vi "Credito Reset.vi"(8 "error in (no error)":errorcluster, 11 "USD Actor in":refnum<class "USD Actor.lvclass">) -> (0 "error out":errorcluster, 3 "USD Actor out":refnum<class "USD Actor.lvclass">)   [LabVIEW 2020, in "USD Actor.lvlib" / "USD Actor.lvclass"]
uses:
  USD Actor.lvclass
  USD Actor.lvclass/USD Actor.ctl
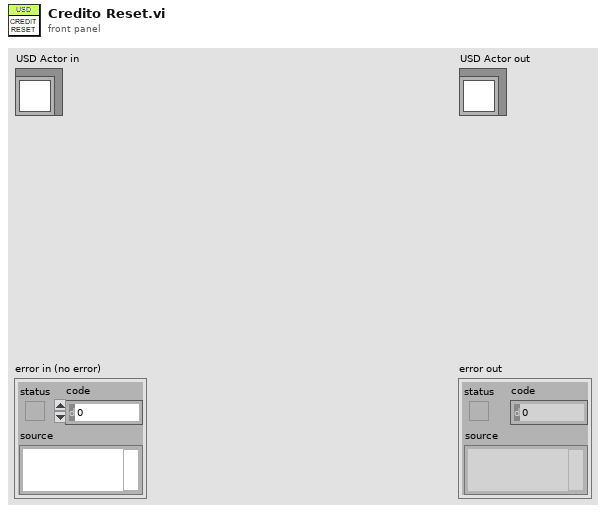
[diagram p1: front panel]
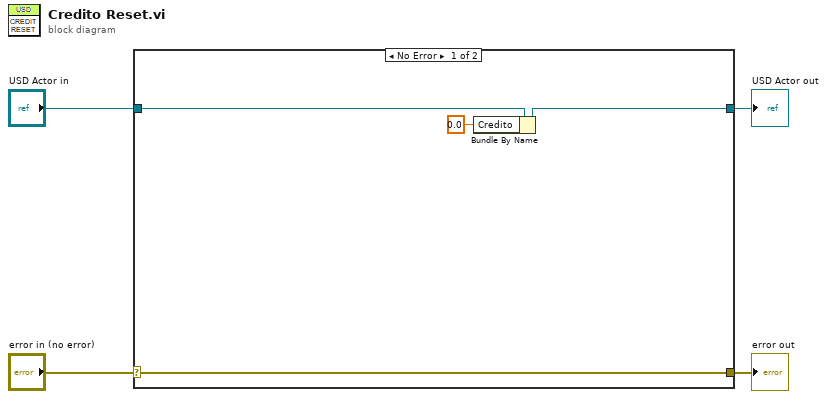
[diagram p0: block diagram]
diagram:
  n1 = case shown="No Error" "error in (no error)" {
    selector: "error in (no error)" -> [w8 w10]
    tunnel: [w8 w10] -> w3
    tunnel: [w6 w9] -> w1
    tunnel: "USD Actor in" -> [w7 w9]
    frame No Error {
      n2 = Bundle By Name(cluster=w7, "Credito"=0.0) -> (w6:refnum<class "USD Actor.lvclass">)
    }
    frame Error {
    }
  }
  "error out" <- w3
  "USD Actor out" <- w1
